vi "Send Direct Command.vi"(0 "Dynamixel Motor in":refnum<class "Dynamixel Motor.lvclass">, 5 "Motor ID (0)":u8, 7 "Address":u8, 9 "Select Action":u16(ring) items=["Ping", "Read", "Write", "Registered Write", "Action", "Reset", "Sync Write"], 11 "error in (no error)":errorcluster, 12 "Parameters":string) -> (4 "Dynamixel Motor out":refnum<class "Dynamixel Motor.lvclass">, 6 "Command to Serial":string, 15 "error out":errorcluster)   [LabVIEW 2016, in "Dynamixel Motor.lvclass"]
doc: "Using any of the six basic commands for the Dynamixel motor, this VI allows you to send any set of parameters to the motor(s). This is a Low-Level VI that is used by other VIs."
uses:
  <instrlib>/Dynamixel Motor/HAIOL/Dynamixel Motor.lvclass
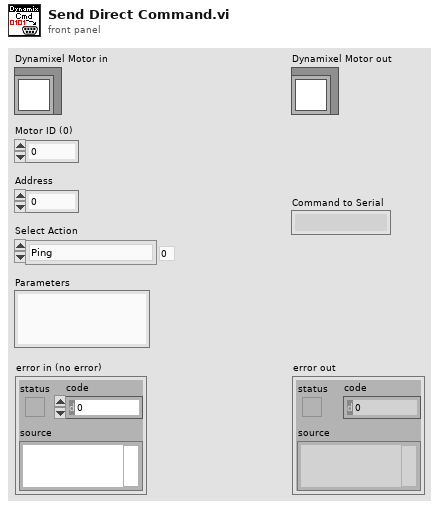
[diagram p1: front panel]
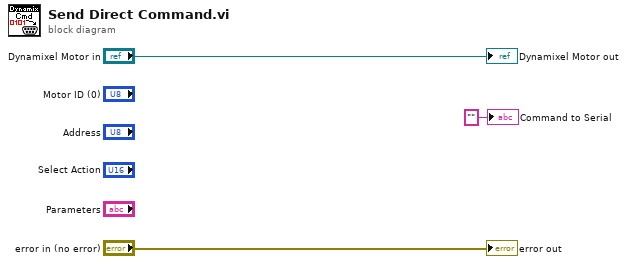
[diagram p0: block diagram]
diagram:
  "error out" <- "error in (no error)"
  "Dynamixel Motor out" <- "Dynamixel Motor in"
  "Command to Serial" <- "" ("Command to Serial")
